vi "uc480_Error_Handling.vi"(9 "Error Code":i32, 10 "Error String":string, 11 "Error In":errorcluster) -> (3 "Error Out":errorcluster)   [LabVIEW 2021]
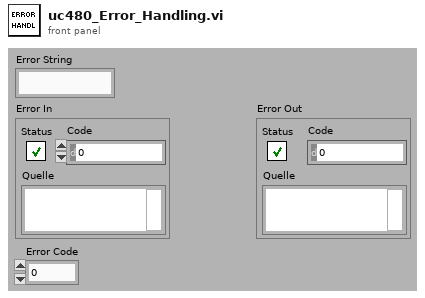
[diagram p1: front panel]
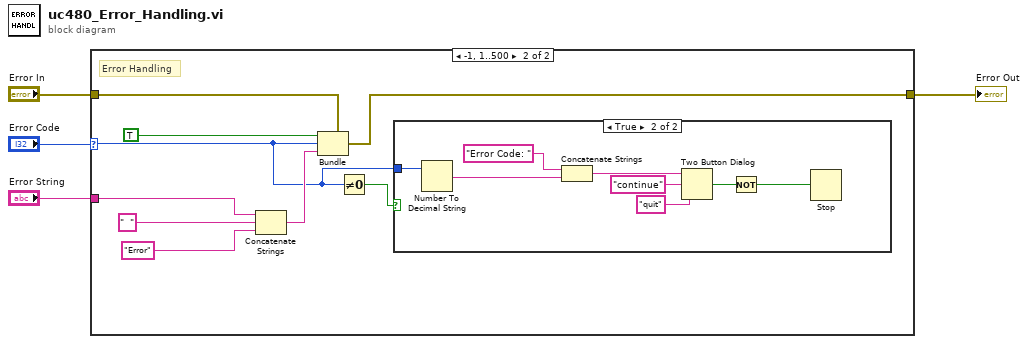
[diagram p0: block diagram]
diagram:
  n1 = case shown="-1, 1..500" "Error Code" {
    selector: "Error Code" -> [_ w6]
    tunnel: "Error In" -> [w5 w14]
    tunnel: [w5 w13] -> w3
    tunnel: "Error String" -> [_ w8]
    frame 0, Default {
      # "Error Handling"
    }
    frame -1, 1..500 {
      # "Error Handling"
      n2 = Concatenate Strings(w8, "  ", "Error") -> (w11:string)
      n3 = Bundle(cluster=w14, "status"=TRUE, "code"=w6, "source"=w11) -> (w13:errorcluster)
      n4 = Not Equal To 0?(x=w6) -> (x != 0?=w7:bool)
      n5 = case shown="True" w7 {
        tunnel: w6 -> [_ w22]
        frame False {
        }
        frame True {
          n6 = Number To Decimal String(number=w22) -> (decimal integer string=w21:string)  [unwired: 1 in]
          n7 = Concatenate Strings("Error Code: " ("string"), w21) -> (w19:string)
          n8 = Two Button Dialog(message=w19, 1:"quit" ("F button name (\"Cancel\")"), 2:"continue" ("T button name (\"OK\")")) -> (T button?=w16:bool)
          n9 = Not(x=w16) -> (.not. x?=w15:bool)
          n10 = Stop(stop? (T)=w15) -> ()
        }
      }
    }
  }
  "Error Out" <- w3
